vi "Interface.vi"(9 "EventsIn":T2, 10 "Events":T3) -> ()   [LabVIEW 2014, in "BuildSpecEditor.lvlib" / "EXESpecEditor.lvclass"]
uses:
  EXESpecEditor.lvclass
  GCMCore/Providers/Veritech_GCM/Support/Framework/_Plugins/_LVCMPlugin/GCMPlugin_EventsOut.ctl
  GCMCore/Providers/Veritech_GCM/Support/Framework/_Plugins/_LVCMPlugin/GCMPlugin_EventsIn.ctl
  <vilib>/AppBuilder/RW_Project/AB_RW_Project_PropBag_Action.ctl
  GCMCore/Providers/Veritech_GCM/Support/Framework/_Plugins/GCMPlugin/GCMPlugin.lvclass
panel:
  in  "Version":T1
  in  "AutoIncrement":bool caption="Auto-increment?"
  # "Warning: unchecking Auto-increment? doesn't work here. If you want to uncheck it, do it from native properties window."
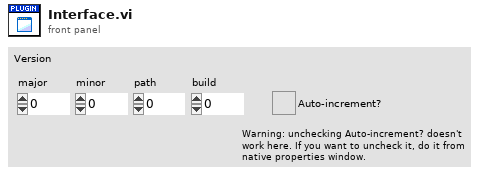
[diagram p1: front panel]
types:
  T1 = cluster{"major":u16, "minor":u16, "path":u16, "build":u16}
  T2 = typedef "GCMPlugin.lvclass/GCMPlugin_EventsIn.ctl" = cluster{"Stop":refnum<user-event>, "ItemSelected":refnum<user-event>, "ItemDeselected":refnum<user-event>, "PluginActivated":refnum<user-event>, "PluginDeactivated":refnum<user-event>}
  T3 = typedef "GCMPlugin.lvclass/GCMPlugin_EventsOut.ctl" = cluster{"ItemEdited":refnum<user-event>}
  T4 = typedef "AB_RW_Project_PropBag_Action.ctl" = enum16{"read", "write", "clear", "readPrevious", "writePrevious", "clearPrevious"}
  T5 = cluster{"Item URL":string, "Item ID":string, "Item Index":i32, "Specific Type":string}
  T6 = typedef "ItemRef.ctl" = u64
  T7 = typedef "AB_RW_Project_Build_Data.ctl" = cluster{"buildSpecName":string, "buildSpecDescription":string, "excludeTypedefs":bool, "excludePolymorphicVIs":bool, "excludeLibraryItems":bool, "modifyLibraryFile":bool, "defaultLanguage":string, "supportedLanguages":string[], "excludedDirectories":path[], "userLog_Path":path, "preActionVIID":string, "postActionVIID":string, "localDest_Path":path, "targetDest_Path":path, "removeVIObject":u16, "previewCache_ID":string, "buildCache_ID":string, "compilerOptimizationLevel":u32, "excludeInlineSubVIs":bool, "bldVersion":cluster{"major":u16, "minor":u16, "patch":u16, "build":u16}, "autoIncrement":bool, "excludeDependentPPLs":bool, "excludeDependentDLLs":bool}
  T8 = cluster{"major":u16, "minor":u16, "patch":u16, "build":u16}
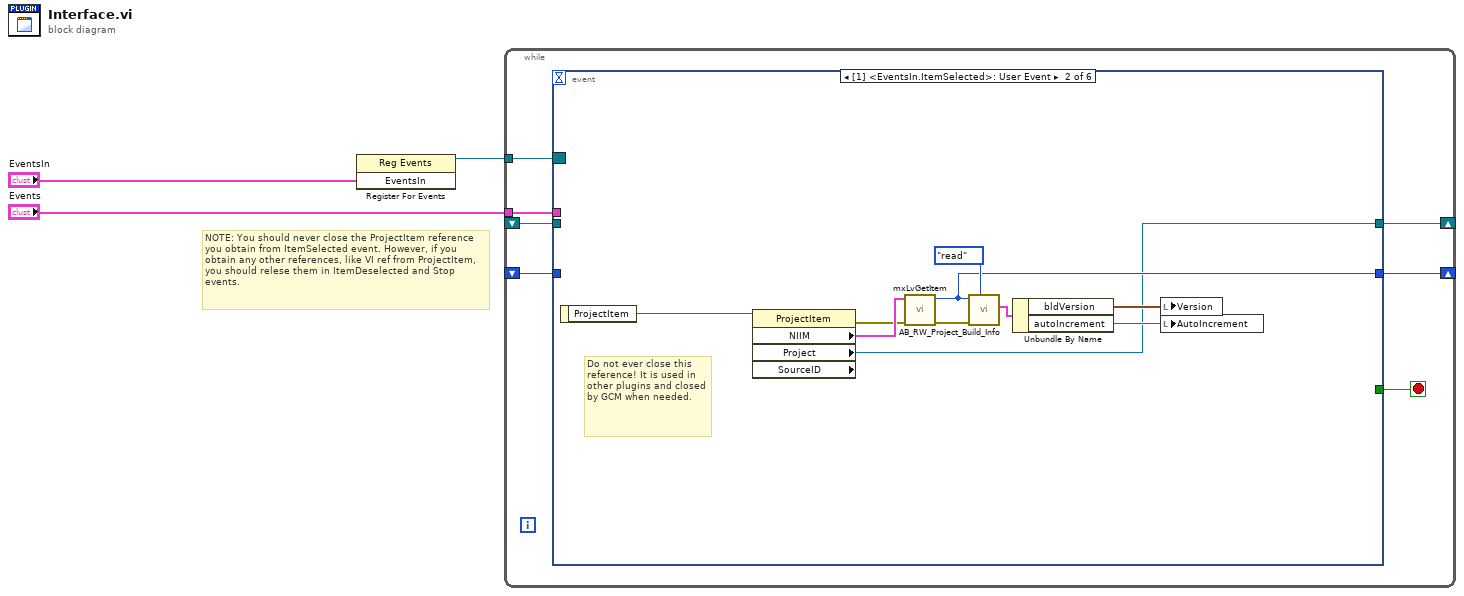
[diagram p0: block diagram]
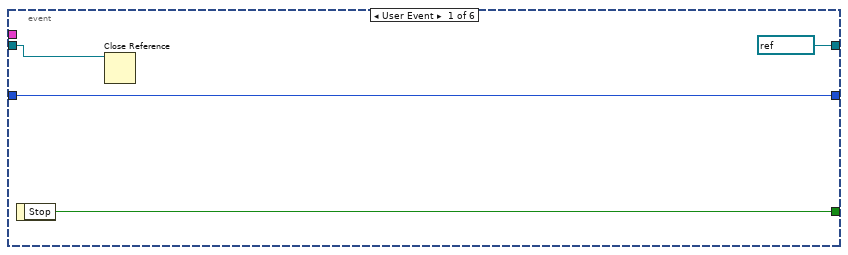
[diagram p2: hidden frame]
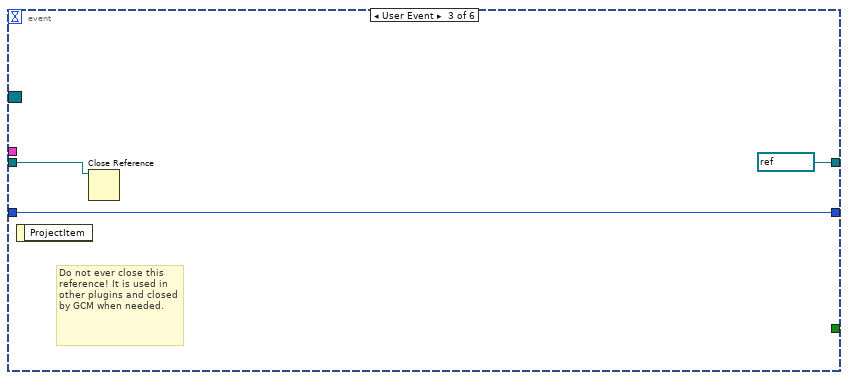
[diagram p3: hidden frame]
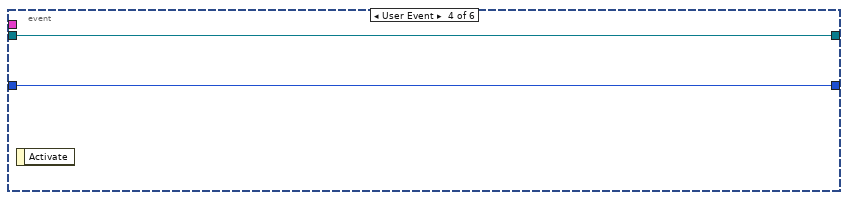
[diagram p4: hidden frame]
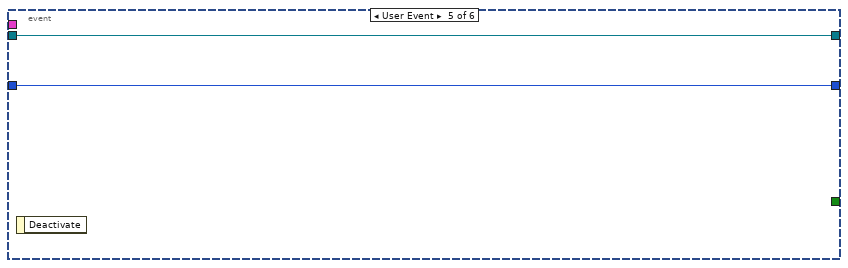
[diagram p5: hidden frame]
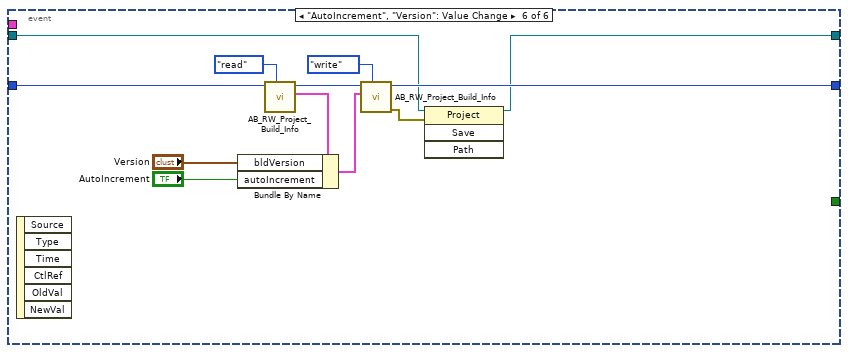
[diagram p6: hidden frame]
diagram:
  # "NOTE: You should never close the ProjectItem reference you obtain from ItemSelected event. However, if you obtain any other references, like VI ref from ProjectItem, you should relese them in ItemDeselected and Stop events."
  n1 = register-events("EventsIn") -> (reference out=w2:refnum<event-registration>)  [unwired: 2 in, 1 out]
  n2 = while {
    tunnel: w2 -> [w10]
    tunnel: "Events" -> [w9]
    shift-right: [w7] -> _
    shift-left: _ -> [w6]
    shift-right: [w5] -> _
    shift-left: _ -> [w4]
    stop <- w8 stop-if-true
    n3 = event shown="[1] <EventsIn.ItemSelected>: User Event" {
      selector: w10 -> [_ _ _ _ _ _]
      dyn-events: _ -> [_ _ _ _ _ _]
      timeout: _ -> [_ _ _ _ _ _]
      tunnel: w9 -> [_ _ _ _ _ _]
      tunnel: [w14 _ _ _ _ _] -> w8
      tunnel: [w13 w20 w27 w29 w31 w42] -> w7
      tunnel: w6 -> [w13 _ w27 w29 w31 w36]
      tunnel: [refnum<vi> refnum ("Project") w16 refnum<vi> refnum ("Project") w28 w30 w39] -> w5
      tunnel: w4 -> [w12 _ w26 w28 w30 w40]
      event User Event {
        n4 = event-data() -> ("Stop"=w14:bool)  [unwired: 1 in]
        n5 = Close Reference(reference=w12) -> ()  [unwired: 1 in, 1 out]
      }
      event User Event {
        # "Do not ever close this reference! It is used in other plugins and closed by GCM when needed."
        n6 = event-data() -> ("ProjectItem"=w15:refnum<vi>)  [unwired: 1 in]
        n7 = property class="ProjectItem" props=["NIIM", "Project", "SourceID"](reference=w15) -> (error out=w21:errorcluster, "NIIM"=w24:T5, "Project"=w16:refnum<vi>)  [unwired: 1 in, 2 out]
        n8 = call <resource>:"mxLvGetItem.vi"("error in"=w21, "NIIM"=w24) -> ("error out"=w22:errorcluster, "Item"=w20:T6)  [unwired: 8 in]
        n9 = call <vilib>:"AB_RW_Project_Build_Info.vi"("action"=AB_RW_Project_PropBag_Action."read", "error in (no error)"=w22, "Object In"=w20) -> ("buildInfo out"=w19:T7)  [unwired: 6 in, 2 out]
        n10 = Unbundle By Name(w19) -> ("bldVersion"=w18:T8, "autoIncrement"=w17:bool)
        n11 = local write "Version"(w18) -> ()
        n12 = local write "AutoIncrement"(w17) -> ()
      }
      event User Event {
        # "Do not ever close this reference! It is used in other plugins and closed by GCM when needed."
        n13 = event-data() -> ()  [unwired: 1 in, 1 out]
        n14 = Close Reference(reference=w26) -> ()  [unwired: 1 in, 1 out]
      }
      event User Event {
        n15 = event-data() -> ()  [unwired: 1 in, 1 out]
      }
      event User Event {
        n16 = event-data() -> ()  [unwired: 1 in, 1 out]
      }
      event "AutoIncrement", "Version": Value Change {
        n17 = event-data() -> ()  [unwired: 1 in, 6 out]
        n18 = call <vilib>:"AB_RW_Project_Build_Info.vi"("action"=AB_RW_Project_PropBag_Action."read", "Object In"=w36) -> ("buildInfo out"=w37:T7, "Object Out"=w35:T6)  [unwired: 7 in, 1 out]
        n19 = Bundle By Name(cluster=w37, "bldVersion"="Version", "autoIncrement"="AutoIncrement") -> (w38:T7)
        n20 = call <vilib>:"AB_RW_Project_Build_Info.vi"("action"=AB_RW_Project_PropBag_Action."write", "buildInfo in"=w38, "Object In"=w35) -> ("error out"=w41:errorcluster, "Object Out"=w42:T6)  [unwired: 6 in, 1 out]
        n21 = invoke class="Project" method="Save"(reference=w40, error in=w41) -> (reference out=w39:refnum<vi>)  [unwired: 2 in, 3 out]
      }
    }
  }
